vi "Get MXN.vi"(8 "error in (no error)":errorcluster, 11 "Soda Actors in":refnum<class "Soda Actors.lvclass">) -> (0 "error out":errorcluster, 2 "MXN":bool, 3 "Soda Actors out":refnum<class "Soda Actors.lvclass">)   [LabVIEW 2020, in "Soda Actors.lvlib" / "Soda Actors.lvclass"]
uses:
  Soda Actors.lvclass
  Soda Actors.lvclass/Soda Actors.ctl
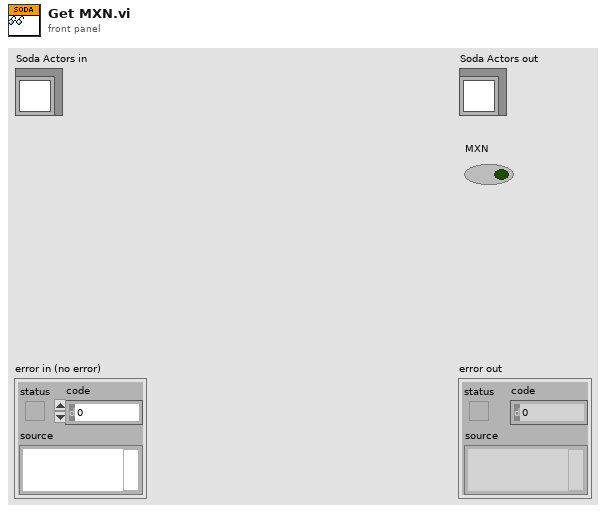
[diagram p1: front panel]
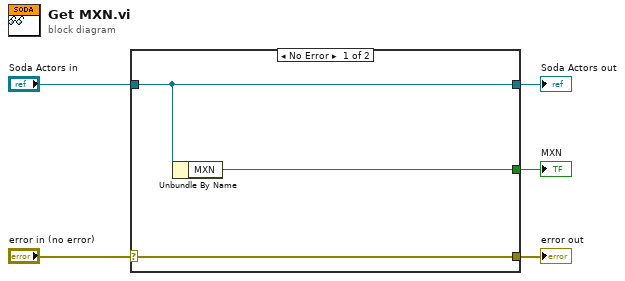
[diagram p0: block diagram]
diagram:
  n1 = case shown="No Error" "error in (no error)" {
    selector: "error in (no error)" -> [w8 w9]
    tunnel: [w8 w9] -> w4
    tunnel: [w7 w10] -> w2
    tunnel: "Soda Actors in" -> [w7 w10]
    tunnel: [w6 _] -> w1
    frame No Error {
      n2 = Unbundle By Name(w7) -> ("MXN"=w6:bool)
    }
    frame Error {
    }
  }
  "error out" <- w4
  "Soda Actors out" <- w2
  "MXN" <- w1
